vi "Mediated_Values.vi"(3 "coda kV/m mediati":refnum<queue>, 4 "coda mV":refnum<queue>) -> (0 "kV/m mediati":string, 1 "mV mediati":string, 2 "4 valori per media\nin array":dbl[](array[numeric]) format="%0.2f")   [LabVIEW 2010]
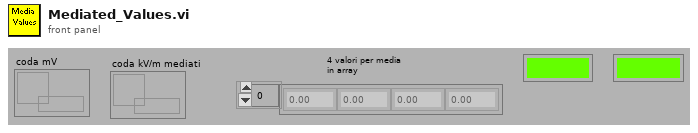
[diagram p1: front panel]
types:
  T1 = cluster{"[0]":dbl, "[1]":dbl, "[2]":dbl, "[3]":dbl, "[4]":dbl, "[5]":dbl, "[6]":dbl, "[7]":dbl, "[8]":dbl}
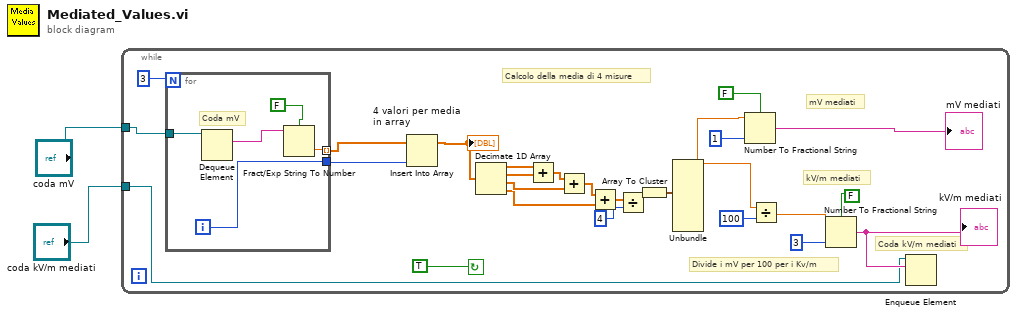
[diagram p0: block diagram]
diagram:
  n1 = while {
    tunnel: "coda mV" -> [w27]
    tunnel: "coda kV/m mediati" -> [w4]
    stop <- TRUE continue-if-true
    # "Coda kV/m mediati"
    # "kV/m mediati"
    # "Divide i mV per 100 per i Kv/m"
    # "mV mediati"
    # "Calcolo della media di 4 misure"
    n2 = for {
      N: 3 -> [_]
      tunnel: [w33] -> w26 mode=indexing
      tunnel: w27 -> [w31]
      tunnel: [w29] -> w25
      i -> [w29]
      # "Coda mV"
      n3 = Dequeue Element(queue=w31) -> (element=w30:string)  [unwired: 2 in, 3 out]
      n4 = Fract/Exp String To Number(use system decimal point (T)=FALSE, string=w30) -> (number=w33:dbl)  [unwired: 2 in, 1 out]
    }
    n5 = Insert Into Array(array=w26, new element=w25) -> (w24:dbl[])  [unwired: 1 in]
    "4 valori per media\nin array" <- w24
    n6 = Decimate 1D Array(w24) -> (w23:dbl[], w22:dbl[], w20:dbl[], w18:dbl[])
    n7 = Add(x=w23, y=w22) -> (x+y=w21:dbl[])
    n8 = Add(x=w21, y=w20) -> (x+y=w19:dbl[])
    n9 = Add(x=w19, y=w18) -> (x+y=w17:dbl[])
    n10 = Divide(x=w17, y=4) -> (x/y=w13:dbl[])
    n11 = Array To Cluster(array=w13) -> (cluster=w12:T1)
    n12 = Unbundle(w12) -> ("[0]"=w8:dbl)  [unwired: 8 out]
    n13 = Number To Fractional String(use system decimal point (T)=FALSE, number=w8, precision (6)=1) -> (F-format string=→"mV mediati":string)  [unwired: 1 in]
    n14 = Divide(x=w8, y=100) -> (x/y=w10:dbl)
    n15 = Number To Fractional String(use system decimal point (T)=FALSE, number=w10, precision (6)=3) -> (F-format string=w5:string)  [unwired: 1 in]
    "kV/m mediati" <- w5
    n16 = Enqueue Element(queue=w4, element=w5) -> ()  [unwired: 2 in, 3 out]
  }
